vi "if_v1_v2.vi"() -> ()   [LabVIEW 2009]
panel:
  out "Rezultat":dbl
  in  "B":dbl
  in  "A":dbl
  in  "Operatia":u16(ring) items=["Adunare", "Scadere", "Inmultire", "Impartire"]
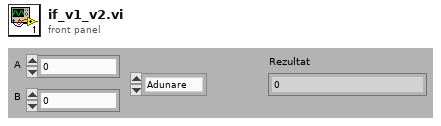
[diagram p1: front panel]
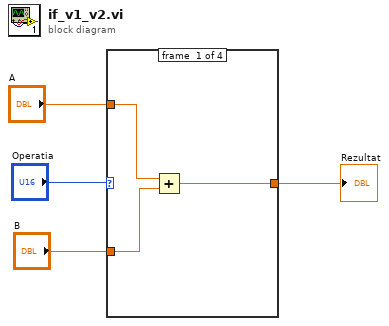
[diagram p0: block diagram]
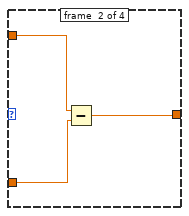
[diagram p2: hidden frame]
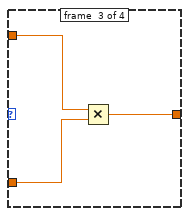
[diagram p3: hidden frame]
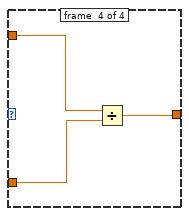
[diagram p4: hidden frame]
diagram:
  n1 = case shown="3" "Operatia" {
    tunnel: "A" -> [w6 w9 w12 w15]
    tunnel: "B" -> [w5 w8 w11 w14]
    tunnel: [w7 w10 w13 w16] -> w1
    frame #0 {
      n2 = Add(x=w6, y=w5) -> (x+y=w7:dbl)
    }
    frame #1 {
      n3 = Subtract(x=w9, y=w8) -> (x-y=w10:dbl)
    }
    frame #2 {
      n4 = Multiply(x=w12, y=w11) -> (x*y=w13:dbl)
    }
    frame #3 {
      n5 = Divide(x=w15, y=w14) -> (x/y=w16:dbl)
    }
  }
  "Rezultat" <- w1
